vi "ex_SetExpAttribsAndT0.vi"(6 "Latch Origin TS? (T)":bool=TRUE, 7 "Set? (T if empty)":bool[](array[boolean]), 8 "error in (no error)":errorcluster, 9 "Express Attributes Plus in":T1[](array[typedef]) {"dX" format="%.2f"; "X0" format="%<%X\n%x>T"; "Timestamp" format="%<%X\n%x>T"; "Start Timestamp" format="%<%X\n%x>T"}, 10 "Origin Timestamps":timestamp[](array[timestamp]) format="%<%X\n%x>T", 11 "Signals":waveform(dbl)[](array[waveform])) -> (0 "error out":errorcluster, 1 "Express Wave Attributes Plus out":T1[](array[typedef]) {"dX" format="%.2f"; "X0" format="%<%X\n%x>T"; "Timestamp" format="%<%X\n%x>T"; "Start Timestamp" format="%<%X\n%x>T"}, 3 "Signals With Attributes":waveform(dbl)[](array[waveform]))   [LabVIEW 2020]
doc: "VI adds all Express waveform attributes to Signals according to inputs Origin Timestamp and Express Attributes. If the input Latch Origin TS? is True, the VI latches the value of Origin Timestamp. When False, the VI applies the stores timestamp from a previous call when True."
uses:
  ex_WaveformAttribs.ctl
  ex_WaveformAttribsPlus.ctl
panel:
  in  "All Express Attributes":T2 {"Timestamp" format="%<%X\n%x>T"; "Start Timestamp" format="%<%X\n%x>T"}
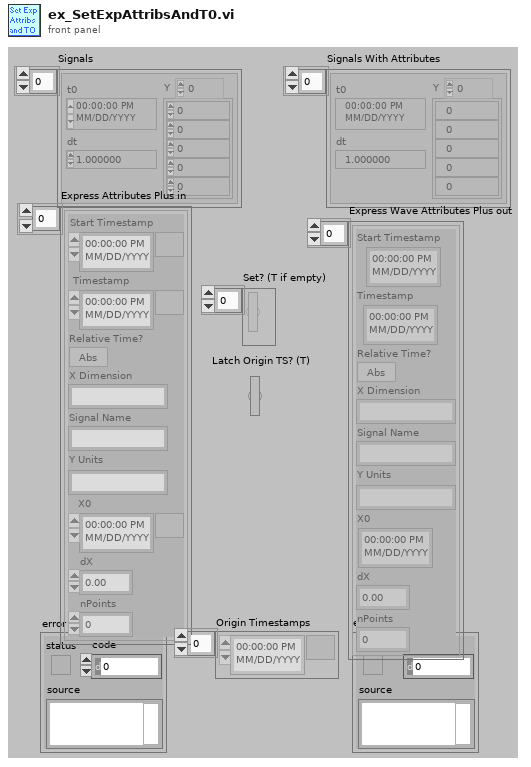
[diagram p1: front panel]
types:
  T1 = typedef "ex_WaveformAttribsPlus.ctl" = cluster{"Start Timestamp":timestamp, "Timestamp":timestamp, "Relative Time?":bool, "X Dimension":string, "Signal Name":string, "Y Units":string, "X0":timestamp, "dX":dbl, "nPoints":i32}
  T2 = typedef "ex_WaveformAttribs.ctl" = cluster{"Start Timestamp":timestamp, "Timestamp":timestamp, "Relative Time?":bool, "X Dimension":string, "Signal Name":string}
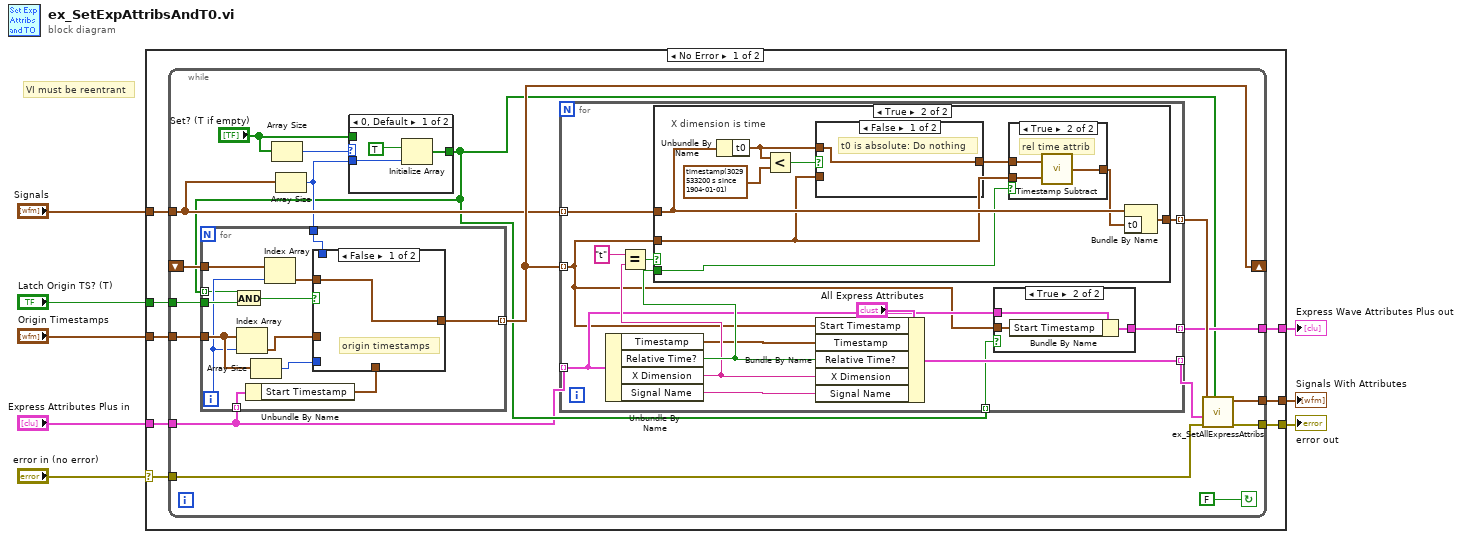
[diagram p0: block diagram]
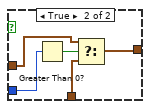
[diagram p2: hidden frame]
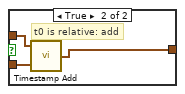
[diagram p7: hidden frame]
diagram:
  # "VI must be reentrant"
  n1 = case shown="No Error" "error in (no error)" {
    selector: "error in (no error)" -> [w12 w95]
    tunnel: [w16 w95] -> w8
    tunnel: [w15 w94] -> w7
    tunnel: "Signals" -> [w14 w94]
    tunnel: "Express Attributes Plus in" -> [w13 w93]
    tunnel: "Latch Origin TS? (T)" -> [w11 _]
    tunnel: [w10 w93] -> w2
    tunnel: "Origin Timestamps" -> [w9 _]
    frame No Error {
      n2 = while {
        tunnel: [w33] -> w16
        tunnel: [w32] -> w15
        tunnel: w14 -> [w21]
        tunnel: w12 -> [w29]
        tunnel: w13 -> [w17]
        shift-right: [w26] -> _
        shift-left: _ -> [w27]
        tunnel: w11 -> [w25]
        tunnel: [w24] -> w10
        tunnel: w9 -> [w23]
        stop <- FALSE continue-if-true
        n3 = Array Size(array="Set? (T if empty)") -> (size(s)=w22:i32)
        n4 = Array Size(array=w21) -> (size(s)=w20:i32)
        n5 = case shown="0, Default" w22 {
          tunnel: w20 -> [w54 _]
          tunnel: "Set? (T if empty)" -> [_ w56]
          tunnel: [w53 w56] -> w18
          frame 0, Default {
            n6 = Initialize Array(TRUE, w54) -> (w53:bool[])
          }
          frame 1.. {
          }
        }
        n7 = for {
          tunnel: w27 -> [w46]
          tunnel: [w45] -> w26 mode=indexing
          tunnel: w25 -> [w44]
          tunnel: w23 -> [w41]
          tunnel: w20 -> [w43]
          tunnel: w18 -> [w36] mode=indexing
          tunnel: w17 -> [w35] mode=indexing
          i -> [w38]
          n8 = And(x=w36, y=w44) -> (x .and. y?=w37:bool)
          n9 = Index Array(array=w41, index=w38) -> (element=w42:timestamp)
          n10 = Unbundle By Name(w35) -> ("Start Timestamp"=w34:timestamp)
          n11 = Array Size(array=w41) -> (size(s)=w40:i32)
          n12 = Index Array(array=w46, index=w38) -> (element=w39:timestamp)
          n13 = case shown="False" w37 {
            tunnel: [w47 w49] -> w45
            tunnel: w39 -> [w47 _]
            tunnel: w42 -> [_ w51]
            tunnel: w43 -> [_ _]
            tunnel: w34 -> [_ w50]
            tunnel: w40 -> [_ w52]
            frame False {
              # "origin timestamps"
            }
            frame True {
              n14 = Greater Than 0?(x=w52) -> (x > 0?=w48:bool)
              n15 = Select(t=w51, s=w48, f=w50) -> (s? t:f=w49:timestamp)
            }
          }
        }
        n16 = for {
          tunnel: [w70] -> w31 mode=indexing
          tunnel: w21 -> [w62] mode=indexing
          tunnel: [w66] -> w30 mode=indexing
          tunnel: w17 -> [w60] mode=indexing
          tunnel: w26 -> [w59] mode=indexing
          tunnel: [w58] -> w24 mode=indexing
          tunnel: w18 -> [w57] mode=indexing
          n17 = Unbundle By Name(w60) -> ("Timestamp"=w61:timestamp, "Relative Time?"=w65:bool, "X Dimension"=w64:string, "Signal Name"=w63:string)
          n18 = Equal?(x="t" ("y"), y=w64) -> (x = y?=w67:bool)
          n19 = case shown="True" w67 {
            tunnel: w59 -> [_ w81]
            tunnel: w65 -> [_ w78]
            tunnel: w62 -> [w75 w82]
            tunnel: [w75 w84] -> w66
            frame False {
              # "X dimension is Not time"
            }
            frame True {
              # "X dimension is time"
              n20 = Unbundle By Name(w82) -> ("t0"=w80:timestamp)
              n21 = Less?(x=w80, y=timestamp(3029533200 s since 1904-01-01) ("number")) -> (x < y?=w79:bool)
              n22 = case shown="False" w79 {
                tunnel: w81 -> [_ w92]
                tunnel: w80 -> [w89 w91]
                tunnel: [w89 w90] -> w76
                frame False {
                  # "t0 is absolute: Do nothing"
                }
                frame True {
                  # "t0 is relative: add"
                  n23 = call "Timestamp Add.vi"("y"=w92, "x"=w91) -> ("x + y"=w90:timestamp)
                }
              }
              n24 = case shown="True" w78 {
                tunnel: w81 -> [_ w88]
                tunnel: w76 -> [w85 w87]
                tunnel: [w85 w86] -> w77
                frame False {
                  # "abs time attrib"
                }
                frame True {
                  # "rel time attrib"
                  n25 = call "Timestamp Subtract.vi"("y"=w88, "x"=w87) -> ("x - y"=w86:timestamp)
                }
              }
              n26 = Bundle By Name(cluster=w82, "t0"=w77) -> (w84:waveform(dbl))
            }
          }
          n27 = Bundle By Name(cluster="All Express Attributes", "Start Timestamp"=w59, "Timestamp"=w61, "Relative Time?"=w65, "X Dimension"=w64, "Signal Name"=w63) -> (w70:T2)
          n28 = case shown="True" w57 {
            tunnel: w60 -> [w71 w74]
            tunnel: w59 -> [_ w73]
            tunnel: [w71 w72] -> w58
            frame False {
            }
            frame True {
              n29 = Bundle By Name(cluster=w74, "Start Timestamp"=w73) -> (w72:T1)
            }
          }
        }
        n30 = call "ex_SetAllExpressAttribs.vi"("Enable (T if empty)"=w18, "error in"=w29, "All Express Wave Attributes"=w31, "Signals"=w30) -> ("error out"=w33:errorcluster, "Signals With Attributes"=w32:waveform(dbl)[])  [unwired: 6 in]
      }
    }
    frame Error {
    }
  }
  "error out" <- w8
  "Signals With Attributes" <- w7
  "Express Wave Attributes Plus out" <- w2
